vi "controlbox_prototype.vi"() -> ()   [LabVIEW 2011]
panel:
  in  "hood man / auton delay":dbl(knob) scale=0.0..10.0
  in  "hood man":bool
  in  "Fold":bool
  in  "Auton":u8(knob) scale=0.0..10.0
  in  "Speed":bool
  in  "Manual":bool
  in  "Manual":dbl(knob) scale=1500.0..2500.0
  in  "Blow":bool
  in  "Force Suck":bool
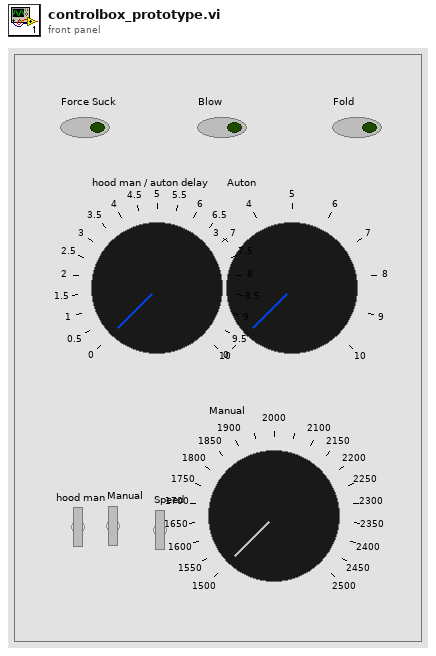
[diagram p1: front panel]
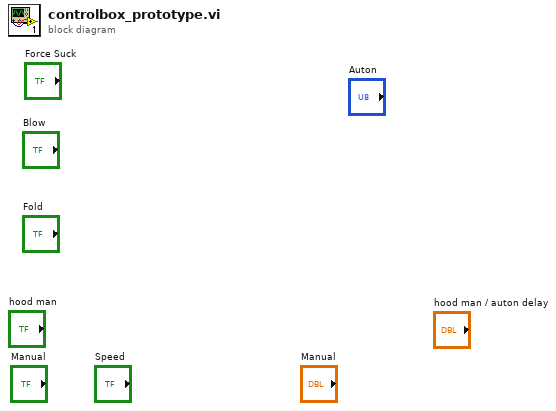
[diagram p0: block diagram]
diagram:
